vi "LOGIC_SendError2Fits.vi"(8 "error in (no error)":errorcluster) -> ()   [LabVIEW 2016]
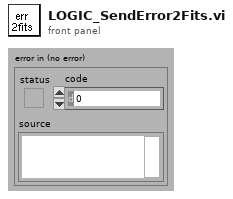
[diagram p1: front panel]
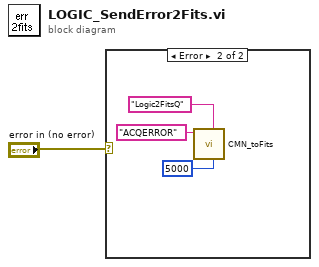
[diagram p0: block diagram]
diagram:
  n1 = case shown="Error" "error in (no error)" {
    frame No Error {
    }
    frame Error {
      n2 = call "CMN_toFits.vi"("ms timeout (-1)"=5000, "response Q"="Logic2FitsQ", "command"="ACQERROR") -> ()  [unwired: 5 in, 4 out]
    }
  }
